vi "ClusterWithNumbersAndStrings.vi"(0 "Cluster":T1={"Numeric"=123.0, "Numeric 2"=456.0+34.0i, "Numeric 3"=789, "String"="Has a default value", "Path"=path "C:/Program Files (x86)/National Instruments/TestStand 4.2.1/Bin/SeqEdit.exe", "Combo Box"="String 1"}, 5 "Which Controls Are Using Default Values":bool[](array[boolean])=[FALSE, FALSE, FALSE, FALSE, FALSE, FALSE]) -> (4 "All Default Values Are Equal":bool)   [LabVIEW 2010]
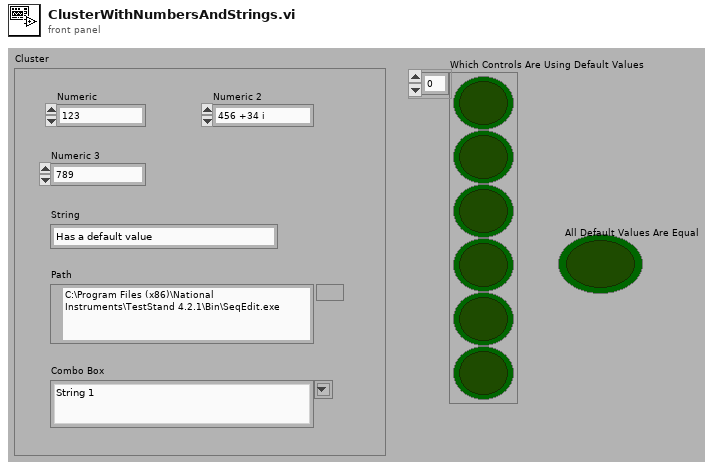
[diagram p1: front panel]
types:
  T1 = cluster{"Numeric":dbl, "Numeric 2":cdb, "Numeric 3":u64, "String":string, "Path":path, "Combo Box":string}
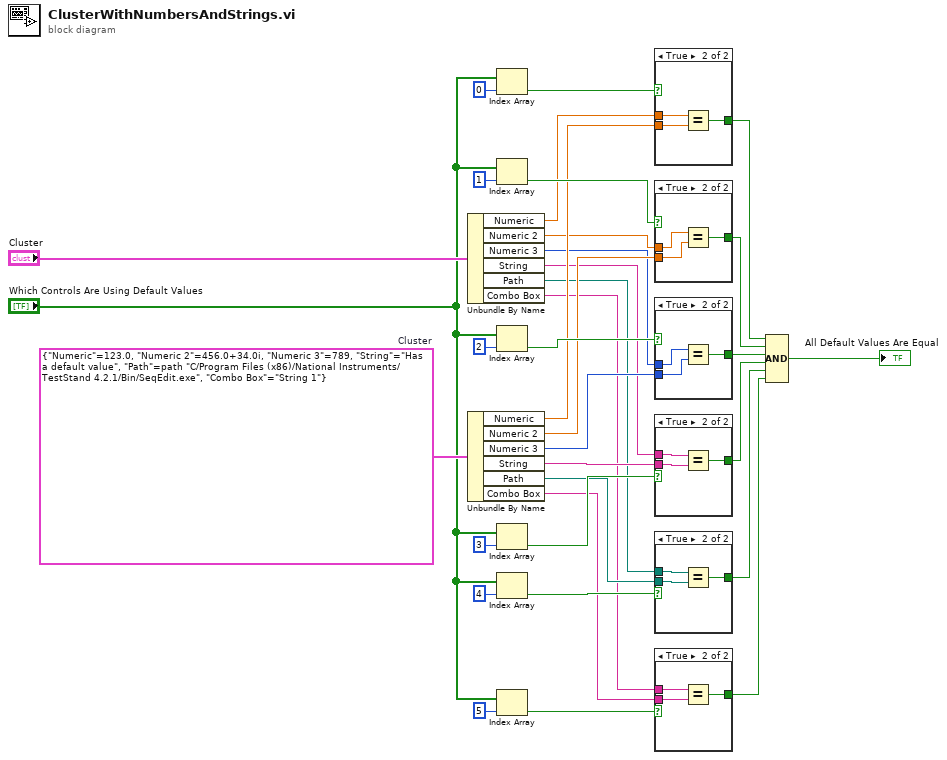
[diagram p0: block diagram]
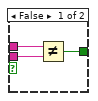
[diagram p2: hidden frame]
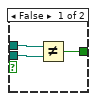
[diagram p3: hidden frame]
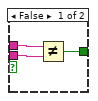
[diagram p4: hidden frame]
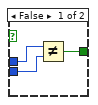
[diagram p5: hidden frame]
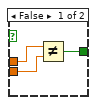
[diagram p6: hidden frame]
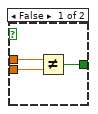
[diagram p7: hidden frame]
diagram:
  w33 = T1 {"Numeric"=123.0, "Numeric 2"=456.0+34.0i, "Numeric 3"=789, "String"="Has a default value", "Path"=path "C:/Program Files (x86)/National Instruments/TestStand 4.2.1/Bin/SeqEdit.exe", "Combo Box"="String 1"}  # Cluster
  n1 = Unbundle By Name("Cluster") -> ("Numeric"=w25:dbl, "Numeric 2"=w16:cdb, "Numeric 3"=w14:u64, "String"=w12:string, "Path"=w10:path, "Combo Box"=w8:string)
  n2 = Unbundle By Name(w33) -> ("Numeric"=w24:dbl, "Numeric 2"=w15:cdb, "Numeric 3"=w13:u64, "String"=w11:string, "Path"=w9:path, "Combo Box"=w7:string)
  n3 = Index Array(array="Which Controls Are Using Default Values", index=0) -> (element=w31:bool)
  n4 = Index Array(array="Which Controls Are Using Default Values", index=1) -> (element=w30:bool)
  n5 = Index Array(array="Which Controls Are Using Default Values", index=2) -> (element=w29:bool)
  n6 = Index Array(array="Which Controls Are Using Default Values", index=3) -> (element=w28:bool)
  n7 = Index Array(array="Which Controls Are Using Default Values", index=4) -> (element=w27:bool)
  n8 = Index Array(array="Which Controls Are Using Default Values", index=5) -> (element=w26:bool)
  n9 = case shown="True" w31 {
    tunnel: w25 -> [w37 w40]
    tunnel: w24 -> [w36 w39]
    tunnel: [w35 w38] -> w23
    frame False {
      n10 = Not Equal?(x=w37, y=w36) -> (x != y?=w35:bool)
    }
    frame True {
      n11 = Equal?(x=w40, y=w39) -> (x = y?=w38:bool)
    }
  }
  n12 = case shown="True" w30 {
    tunnel: [w41 w46] -> w22
    tunnel: w16 -> [w43 w45]
    tunnel: w15 -> [w42 w44]
    frame False {
      n13 = Not Equal?(x=w43, y=w42) -> (x != y?=w41:bool)
    }
    frame True {
      n14 = Equal?(x=w45, y=w44) -> (x = y?=w46:bool)
    }
  }
  n15 = case shown="True" w29 {
    tunnel: [w47 w52] -> w21
    tunnel: w14 -> [w49 w51]
    tunnel: w13 -> [w48 w50]
    frame False {
      n16 = Not Equal?(x=w49, y=w48) -> (x != y?=w47:bool)
    }
    frame True {
      n17 = Equal?(x=w51, y=w50) -> (x = y?=w52:bool)
    }
  }
  n18 = case shown="True" w28 {
    tunnel: [w53 w58] -> w20
    tunnel: w12 -> [w55 w57]
    tunnel: w11 -> [w54 w56]
    frame False {
      n19 = Not Equal?(x=w55, y=w54) -> (x != y?=w53:bool)
    }
    frame True {
      n20 = Equal?(x=w57, y=w56) -> (x = y?=w58:bool)
    }
  }
  n21 = case shown="True" w27 {
    tunnel: [w59 w64] -> w19
    tunnel: w10 -> [w61 w63]
    tunnel: w9 -> [w60 w62]
    frame False {
      n22 = Not Equal?(x=w61, y=w60) -> (x != y?=w59:bool)
    }
    frame True {
      n23 = Equal?(x=w63, y=w62) -> (x = y?=w64:bool)
    }
  }
  n24 = case shown="True" w26 {
    tunnel: [w65 w70] -> w18
    tunnel: w8 -> [w67 w69]
    tunnel: w7 -> [w66 w68]
    frame False {
      n25 = Not Equal?(x=w67, y=w66) -> (x != y?=w65:bool)
    }
    frame True {
      n26 = Equal?(x=w69, y=w68) -> (x = y?=w70:bool)
    }
  }
  n27 = Compound Arithmetic op=AND(w23, w22, w21, w20, w19, w18) -> (→"All Default Values Are Equal":bool)
